vi "init_DIC.vi"(5 "LiCor VISA Ref":refnum<visa-resource-name>="COM11", 6 "Kloehn VISA Ref":refnum<visa-resource-name>="COM10", 7 "Relay VISA Ref":refnum<visa-resource-name>="COM12") -> (0 "LiCor error out":errorcluster, 1 "kloehn error out":errorcluster, 2 "relay error out":errorcluster, 3 "session bundle out":T1={"relay session out"={"VISA resource out"="COM12", "error out"={"status"=FALSE, "code"=0, "source"=""}}, "kloehn session out"={"VISA resource out"="COM12", "error out"={"status"=FALSE, "code"=0, "source"=""}}, "LiCor session out"={"VISA resource out"="COM12", "error out"={"status"=FALSE, "code"=0, "source"=""}}})   [LabVIEW 2010]
panel:
  # "This initializes all of the instruments and gets everything ready for the rest of the application flow."
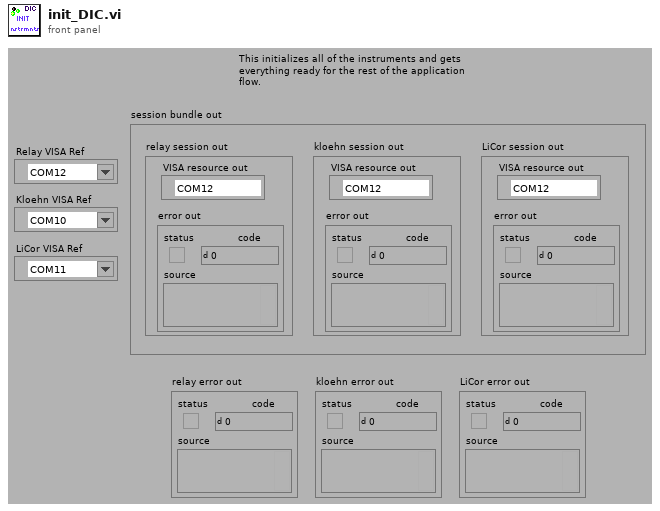
[diagram p1: front panel]
types:
  T1 = cluster{"relay session out":cluster{"VISA resource out":refnum<visa-resource-name>, "error out":errorcluster}, "kloehn session out":cluster{"VISA resource out":refnum<visa-resource-name>, "error out":errorcluster}, "LiCor session out":cluster{"VISA resource out":refnum<visa-resource-name>, "error out":errorcluster}}
  T2 = cluster{"VISA resource out":refnum<visa-resource-name>, "error out":errorcluster}
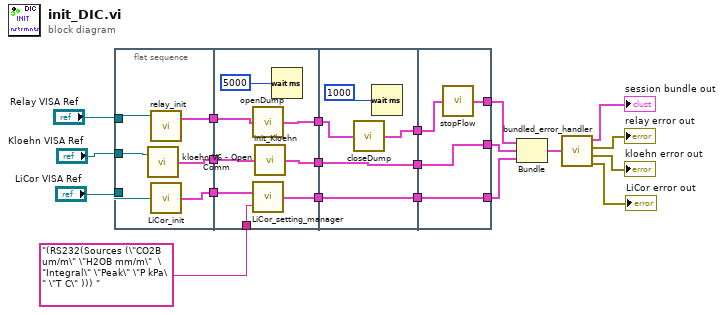
[diagram p0: block diagram]
diagram:
  n1 = flat-sequence {
    tunnel: [w27] -> w21
    tunnel: [w26] -> w20
    tunnel: "Kloehn VISA Ref" -> [w25]
    tunnel: "Relay VISA Ref" -> [w24]
    tunnel: [w23] -> w12
    tunnel: "LiCor VISA Ref" -> [w22]
    tunnel: [w31] -> w19
    tunnel: [w33] -> w18
    tunnel: w21 -> [w34]
    tunnel: w20 -> [w32]
    tunnel: "(RS232(Sources (\"CO2B um/m\" \"H2OB mm/m\"  \"Integral\" \"Peak\" \"P kPa\" \"T C\" ))) " ("String") -> [w30]
    tunnel: w12 -> [w29]
    tunnel: [w28] -> w10
    tunnel: w19 -> [w39]
    tunnel: [w39] -> w17
    tunnel: w18 -> [w38]
    tunnel: [w37] -> w16
    tunnel: [w36] -> w11
    tunnel: w10 -> [w36]
    tunnel: w17 -> [w44]
    tunnel: [w44] -> w7
    tunnel: w16 -> [w43]
    tunnel: [w42] -> w8
    tunnel: [w41] -> w6
    tunnel: w11 -> [w41]
    frame #0 {
      n2 = call "kloehn V6 - Open Comm .vi"("VISA Ref in"=w25) -> ("kloehn  session out"=w26:T2)  [unwired: 1 in]
      n3 = call "relay_init.vi"("VISA resource in"=w24) -> ("relay session out"=w27:T2)  [unwired: 3 in]
      n4 = call "LiCor_init.vi"("VISA resource name"=w22) -> ("LiCor session out"=w23:T2)
    }
    frame #1 {
      n5 = call "openDump.vi"("relay session in"=w34) -> ("relay session out"=w33:T2)
      n6 = call "LiCor_setting_manager.vi"("string to write"=w30, "LiCor session in"=w29) -> ("LiCor session out"=w28:T2)
      n7 = call "init_Kloehn.vi"("kloehn session in"=w32) -> ("kloehn session out"=w31:T2)
      n8 = Wait (ms)(milliseconds to wait=5000) -> ()  [unwired: 1 out]
    }
    frame #2 {
      n9 = call "closeDump.vi"("relay session in"=w38) -> ("relay session out"=w37:T2)
      n10 = Wait (ms)(milliseconds to wait=1000) -> ()  [unwired: 1 out]
    }
    frame #3 {
      n11 = call "stopFlow.vi"("relay session in"=w43) -> ("relay session out"=w42:T2)
    }
  }
  n12 = Bundle("relay session out"=w8, "kloehn session out"=w7, "LiCor session out"=w6) -> (w5:T1)  [unwired: 1 in]
  n13 = call "bundled_error_handler.vi"("session bundle in"=w5) -> ("LiCor error out"=→"LiCor error out":errorcluster, "kloehn error out"=→"kloehn error out":errorcluster, "relay error out"=→"relay error out":errorcluster, "session bundle out"=→"session bundle out":T1)  [unwired: 7 in]
